vi "Line Follower PID Fwd Dis.vi"(5 "Threshold to stop":i32=1200, 6 "Target reflection":sgl, 7 "Threshold to swtich":i32=1200, 8 "Threshold to slow":i32=1000, 9 "Min. speed":i32=40, 10 "Max. speed":i32=80, 11 "EV3 in":T1) -> (3 "EV3 out":T1)   [LabVIEW 2016]
uses:
  <vilib>/NXT/Subs/LVHSConnector.ctl
  <vilib>/NXT/LegoClasses/BrickReference/BrickReference.lvclass
  <vilib>/NXT/Block Support/NXT_OutputPort.ctl
  <vilib>/NXT/NXTIO Xnodes/NXTIONodeSubVIs/LEGOResetMotors.vi
  <vilib>/NXT/Dual Mode Library/Motors/Rotation.vi
  <vilib>/NXT/NXTIO Xnodes/NXTIONodeSubVIs/NXTMotorSteeringOn.vi
  <vilib>/NXT/NXTIO Xnodes/NXTIONodeSubVIs/NXTStopMotors.vi
  <vilib>/NXT/Dual Mode Library/Waits/Wait_Num.vi
  <vilib>/NXT/NXTIO Xnodes/NXTIOXNode/NXTIO.xnode
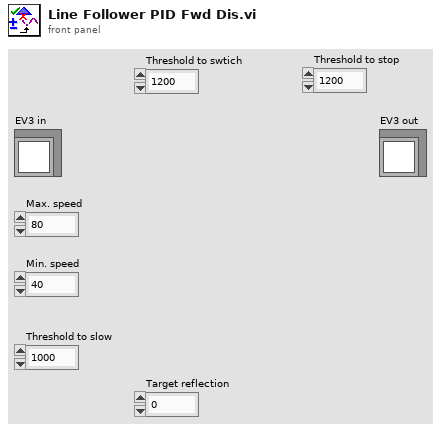
[diagram p1: front panel]
types:
  T1 = typedef "LVHSConnector.ctl" = refnum<class "BrickReference.lvclass">
  T2 = typedef "NXT_OutputPort.ctl" = u8
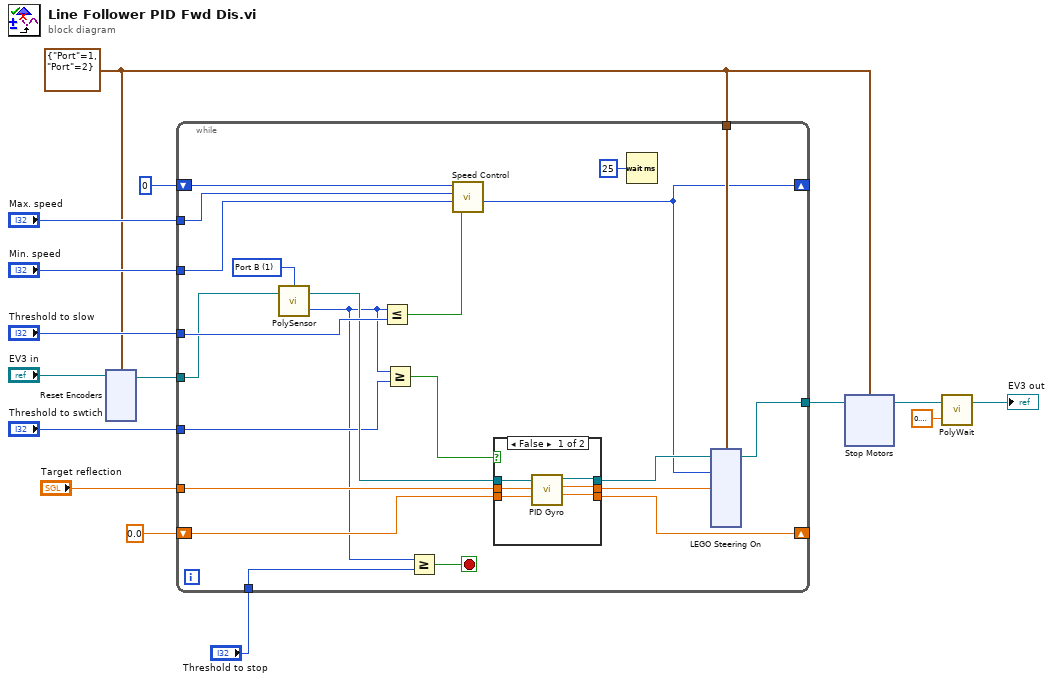
[diagram p0: block diagram]
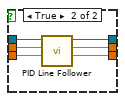
[diagram p2: hidden frame]
diagram:
  w5 = cluster{"Port":T2, "Port":T2} {"Port"=1, "Port"=2} ("Motor")
  n1 = xnode "Reset Encoders"("Motors"=w5, "NXT/EV3"="EV3 in") -> ("NXT/EV3"=w11:T1)
  n2 = while {
    tunnel: w11 -> [w29]
    shift-right: [w20] -> _
    shift-left: sgl 0.0 -> [w22]
    tunnel: "Target reflection" -> [w23]
    tunnel: [w35] -> w7
    tunnel: w5 -> [w37]
    shift-right: [w25] -> _
    shift-left: 0 -> [w33]
    tunnel: "Min. speed" -> [w30]
    tunnel: "Max. speed" -> [w32]
    tunnel: "Threshold to slow" -> [w31]
    tunnel: "Threshold to swtich" -> [w24]
    tunnel: "Threshold to stop" -> [w17]
    stop <- w18 stop-if-true
    w36 = T2 1 items=["Port A", "Port B", "Port C", "Port D"] ("Port (Port A)")
    n3 = call-poly <vilib>:"PolySensor.vi"("NXT/EV3"=w29, "Port (Port A)"=w36) -> ("Angle of Rotation"=w16:i32, "NXT/EV3"=w28:T1)  [unwired: 1 in]
    n4 = Less Or Equal?(x=w16, y=w31) -> (x <= y?=w27:bool)
    n5 = Greater Or Equal?(x=w16, y=w24) -> (x >= y?=w19:bool)
    n6 = Greater Or Equal?(x=w16, y=w17) -> (x >= y?=w18:bool)
    n7 = call "Speed Control.vi"("Speed Up or Down?"=w27, "Min. speed"=w30, "Max. speed"=w32, "Ini. speed"=w33) -> ("Speed out"=w25:i32)  [unwired: 7 in]
    n8 = case shown="False" w19 {
      tunnel: w28 -> [w43 w49]
      tunnel: [w40 w48] -> w26
      tunnel: w23 -> [w42 w47]
      tunnel: w22 -> [w41 w46]
      tunnel: [w39 w45] -> w21
      tunnel: [w38 w44] -> w20
      frame False {
        n9 = call "PID Gyro.vi"("Previous integral"=w41, "Target angle"=w42, "EV3 in"=w43) -> ("New integral"=w38:sgl, "Total error"=w39:sgl, "EV3 out"=w40:T1)  [unwired: 6 in]
      }
      frame True {
        n10 = call "PID Line Follower.vi"("Previous integral\nerror"=w46, "Target reflection"=w47, "EV3 in"=w49) -> ("New integral"=w44:sgl, "Total error"=w45:sgl, "EV3 out"=w48:T1)  [unwired: 6 in]
      }
    }
    n11 = Wait (ms)(milliseconds to wait=u32 25) -> ()  [unwired: 1 out]
    n12 = xnode "LEGO Steering On"("Steering 1"=w21, "Power 1"=w25, "Motors"=w37, "NXT/EV3"=w26) -> ("NXT/EV3"=w35:T1)
  }
  n13 = xnode "Stop Motors"("Motors"=w5, "NXT/EV3"=w7) -> ("NXT/EV3"=w6:T1)
  n14 = call-poly <vilib>:"PolyWait.vi"("Time (1 sec)"=sgl 0.2, "NXT/EV3"=w6) -> ("NXT/EV3"=→"EV3 out":T1)  [unwired: 2 in]
